vi "Init listbox.vi"(8 "error in (no error)":errorcluster, 11 "MulticolumnListbox in":refnum<vi>) -> (0 "error out":errorcluster)   [LabVIEW 2014]
uses:
  <vilib>/Utility/miscctls.llb/LVRowAndColumnUnsignedTypeDef.ctl
  <vilib>/Utility/miscctls.llb/LVRowAndColumnTypeDef.ctl
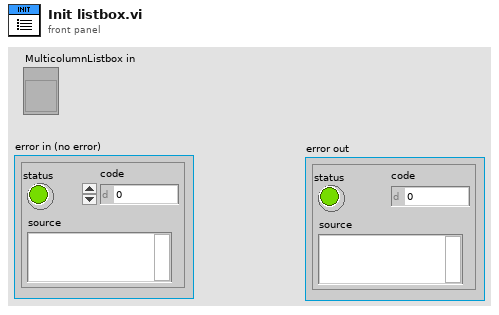
[diagram p1: front panel]
types:
  T1 = typedef "LVRowAndColumnUnsignedTypeDef.ctl" = cluster{"Row":u32, "Column":u32}
  T2 = typedef "LVRowAndColumnTypeDef.ctl" = cluster{"Row":i32, "Column":i32}
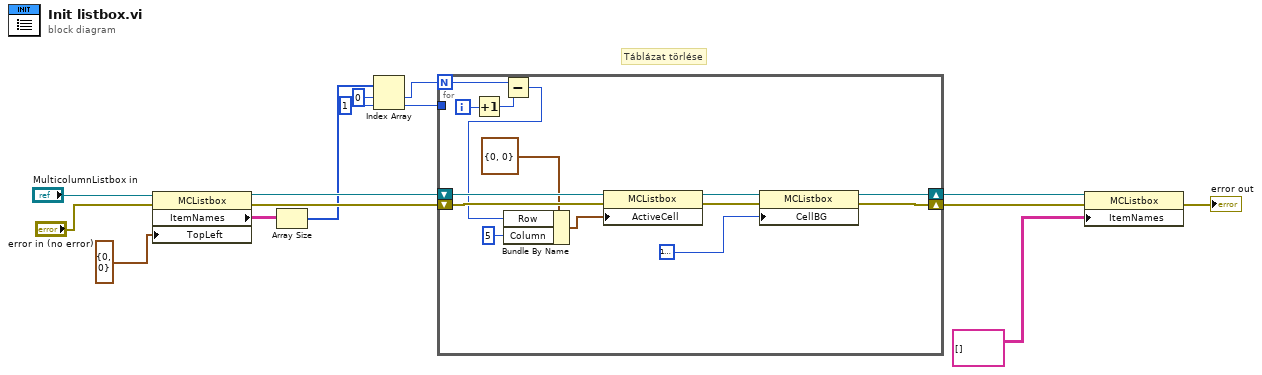
[diagram p0: block diagram]
diagram:
  # "Táblázat törlése"
  n1 = property class="MCListbox"(reference="MulticolumnListbox in", error in="error in (no error)", "TopLeft"=T1 {"Row"=0, "Column"=0} ("Top Left Visible Cell")) -> (reference out=w10:refnum<vi>, error out=w9:errorcluster, "ItemNames"=w3:string[][])
  n2 = Array Size(array=w3) -> (size(s)=w8:i32[])
  n3 = Index Array(array=w8, index #1=0 ("index"), index #2=1 ("index")) -> (element #1=w5:i32, element #2=w4:i32)
  n4 = for {
    N: w5 -> [w19]
    shift-right: [w27] -> w14
    shift-left: w9 -> [w28]
    tunnel: w4 -> [_]
    shift-right: [w26] -> w11
    shift-left: w10 -> [w29]
    i -> [w17]
    n5 = Increment(x=w17) -> (x+1=w16:i32)
    n6 = Subtract(x=w19, y=w16) -> (x-y=w18:i32)
    n7 = Bundle By Name(cluster=T2 {"Row"=0, "Column"=0} ("Active Cell:Active Cell"), "Row"=w18, "Column"=5) -> (w25:T2)
    n8 = property class="MCListbox"(reference=w29, error in=w28, "ActiveCell"=w25) -> (reference out=w22:refnum<vi>, error out=w23:errorcluster)
    n9 = property class="MCListbox"(reference=w22, error in=w23, "CellBG"=u32 16777226) -> (reference out=w26:refnum<vi>, error out=w27:errorcluster)
  }
  n10 = property class="MCListbox"(reference=w11, error in=w14, "ItemNames"=string[][] []) -> (error out=→"error out":errorcluster)  [unwired: 1 out]
